vi "getHueSatInt.vi"(6 "Fiber Num":i32, 8 "Error":bool, 9 "VISA resource name":refnum<visa-resource-name>="ASRL13::INSTR") -> (0 "Saturation":u32, 1 "Hue":dbl, 2 "Error":bool, 3 "dup VISA resource name":refnum<visa-resource-name>="ASRL13::INSTR", 4 "Intensity":u32)   [LabVIEW 2020, in "Library Instrument & Equipement.lvlib" / "Library LED Analyser.lvlib"]
uses:
  Library LED Analyser.lvlib
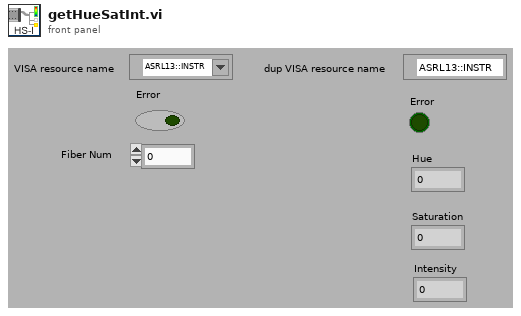
[diagram p1: front panel]
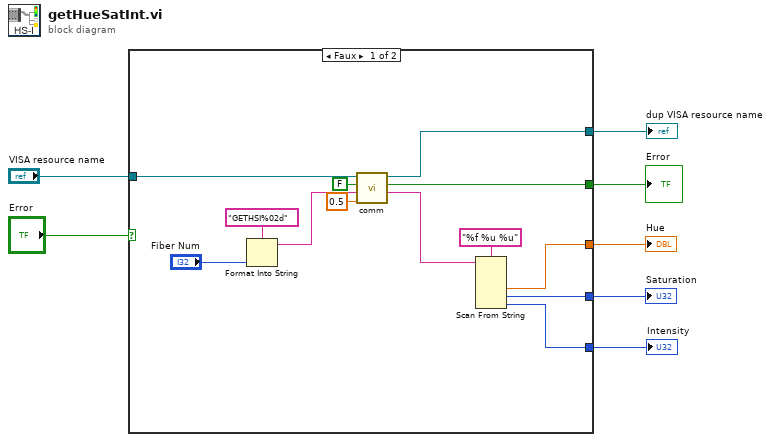
[diagram p0: block diagram]
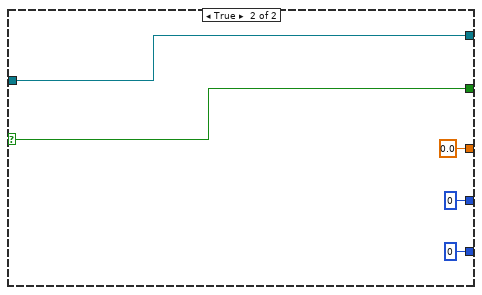
[diagram p2: hidden frame]
diagram:
  n1 = case shown="Faux" "Error" {
    selector: "Error" -> [_ w25]
    tunnel: "VISA resource name" -> [w20 w24]
    tunnel: [w18 0.0] -> w6
    tunnel: [w17 0] -> w5
    tunnel: [w16 0] -> w4
    tunnel: [w12 w24] -> w3
    tunnel: [w11 w25] -> w2
    frame False {
      n2 = Format Into String(format string="GETHSI%02d" ("Substring"), "Fiber Num") -> (resulting string=w13:string)  [unwired: 2 in, 1 out]
      n3 = call "comm.vi"("Timeout (s)"=0.5, "Command"=w13, "Error"=FALSE, "VISA resource name"=w20) -> ("Response"=w10:string, "Error"=w11:bool, "dup VISA resource name"=w12:refnum<visa-resource-name>)  [unwired: 2 in, 1 out]
      n4 = Scan From String(format string="%f %u %u", input string=w10) -> (output 1=w18:dbl, output 2=w17:u32, output 3=w16:u32)  [unwired: 5 in, 3 out]
    }
    frame True {
    }
  }
  "dup VISA resource name" <- w3
  "Error" <- w2
  "Saturation" <- w5
  "Hue" <- w6
  "Intensity" <- w4
